vi "GetAttributeViInt32_SE_SpE_Trigger_OB.vi"(8 "error in (no error)":errorcluster {"code" format="%.0x"}, 9 "AttributeID":u32(ring)=1190055 items=["OCCUPIED_BANDWIDTH_AVERAGE_COUNT"=1190055, "OCCUPIED_BANDWIDTH_AVERAGE_MODE"=1190389, "OCCUPIED_BANDWIDTH_DETECTOR_TYPE"=1190567, "OCCUPIED_BANDWIDTH_DISPLAY_BOUNDARY_FREQUENCY_DISPLAY_TYPE"=1191461, "OCCUPIED_BANDWIDTH_DISPLAY_REF_POSITION"=1190662, "OCCUPIED_BANDWIDTH_DISPLAY_VIEW"=1191462, "OCCUPIED_BANDWIDTH_DISPLAY_VIEW_SELECTION"=1191463, "OCCUPIED_BANDWIDTH_MARKER_ACTIVE_MARKER"=1190395, "OCCUPIED_BANDWIDTH_MARKER_COUNT"=1190397, "OCCUPIED_BANDWIDTH_MARKER_DELTA_REFERENCE"=1190398, "OCCUPIED_BANDWIDTH_MARKER_TYPE"=1190568, "OCCUPIED_BANDWIDTH_POWER_REFERENCE_TYPE"=1191568, "OCCUPIED_BANDWIDTH_SWEEPCOUPLING_BANDWIDTH_SHAPE"=1190408, "OCCUPIED_BANDWIDTH_SWEEPCOUPLING_SWEEP_POINTS"=1190411, "OCCUPIED_BANDWIDTH_SWEEPCOUPLING_SWEEP_TIME_AUTO_RULES"=1190416, "OCCUPIED_BANDWIDTH_TRACE_COUNT"=1150708, "OCCUPIED_BANDWIDTH_TRACE_TYPE"=1150063, "OCCUPIED_BANDWIDTH_TRIGGER_SOURCE"=1150039, "SEMASK_AVERAGE_COUNT"=1190069, "SEMASK_DISPLAY_VIEW"=1190492, "SEMASK_DISPLAY_VIEW_SELECTION"=1150114, "SEMASK_DISPLAY_WINDOWX_REF_POSITION"=1191467, "SEMASK_DISPLAY_WINDOWY_REF_POSITION"=1190664, "SEMASK_MARKER_ACTIVE_MARKER"=1190493, "SEMASK_MARKER_COUNT"=1190495, "SEMASK_MARKER_TYPE"=1190584, "SEMASK_MEASUREMENT_TYPE"=1190475, "SEMASK_OFFSET_AVERAGE_TYPE"=1191572, "SEMASK_OFFSET_DETECTOR_TYPE"=1190508, "SEMASK_REFERENCE_CHANNEL_AVERAGE_TYPE"=1191571, "SEMASK_REFERENCE_CHANNEL_DETECTOR_TYPE"=1190485, "SEMASK_REFERENCE_CHANNEL_SWEEP_TYPE"=1191472, "SEMASK_REFERENCE_CHANNEL_SWEEP_TYPE_AUTO_RULES"=1191474, "SEMASK_SWEEPCOUPLING_BANDWIDTH_SHAPE"=1150117, "SEMASK_TRACE_COUNT"=1150710, "SEMASK_TRACE_TYPE"=1150115, "SEMASK_TRIGGER_SOURCE"=1150062, "SPECIFIC_DRIVER_CLASS_SPEC_MAJOR_VERSION"=1050515, "SPECIFIC_DRIVER_CLASS_SPEC_MINOR_VERSION"=1050516, "SPURIOUS_EMISSIONS_AVERAGE_COUNT"=1190516, "SPURIOUS_EMISSIONS_AVERAGE_MODE"=1190518, "SPURIOUS_EMISSIONS_DISPLAY_VIEW_SELECTION"=1191486, "SPURIOUS_EMISSIONS_DISPLAY_VIEW"=1190669, "SPURIOUS_EMISSIONS_MARKER_ACTIVE_MARKER"=1190523, "SPURIOUS_EMISSIONS_MARKER_COUNT"=1190525, "SPURIOUS_EMISSIONS_MARKER_DELTA_REFERENCE"=1190527, "SPURIOUS_EMISSIONS_MARKER_TYPE"=1190533, "SPURIOUS_EMISSIONS_MEASUREMENT_TYPE"=1190509, "SPURIOUS_EMISSIONS_REPORT_MODE"=1190514, "SPURIOUS_EMISSIONS_SWEEP_TIME_AUTO_RULE"=1150125, "SPURIOUS_EMISSIONS_TRIGGER_SOURCE"=1150068, "SPURIOUSEMISSIONSTRACE_COUNT"=1190614, "SWEEP_TIME_AUTO_RULES"=1191711, "SYSTEM_IO_TIMEOUT"=1191768, "TRIGGER_AIQ_MAGNITUDE_SLOPE"=1190819, "TRIGGER_EXTERNAL2_SLOPE"=1190145, "TRIGGER_EXTERNAL_SLOPE"=1190141, "TRIGGER_FRAME_SYNC_SOURCE"=1190149, "TRIGGER_FRAME_SYNCHOLDOFF_TYPE"=1150129, "TRIGGER_I_DEMODULATED_SLOPE"=1190823, "TRIGGER_INPUT_I_SLOPE"=1190827, "TRIGGER_INPUT_Q_SLOPE"=1190839, "TRIGGER_IQ_MAGNITUDE_SLOPE"=1190831, "TRIGGER_LINE_SLOPE"=1190160, "TRIGGER_Q_DEMODULATED_SLOPE"=1190835, "TRIGGER_RFBURST_LEVEL_TYPE"=1190166, "TRIGGER_RFBURST_SLOPE"=1190163, "TRIGGER_VIDEO_SLOPE"=1190170], 10 "RepCapIdentifier":string, 11 "instrument handle":refnum<k15>) -> (0 "error out":errorcluster {"code" format="%.0x"}, 2 "AttributeValue":i32, 3 "instrument handle out":refnum<k15>)   [LabVIEW 2021, in "Keysight XSAnVMA.lvlib"]
doc: "Gets Int32 Attribute from instrumrnt driver.\nThe following attributes are supported:\n\nOCCUPIED_BANDWIDTH_AVERAGE_COUNT\nOCCUPIED_BANDWIDTH_AVERAGE_MODE\nOCCUPIED_BANDWIDTH_DETECTOR_TYPE\nOCCUPIED_BANDWIDTH_DISPLAY_BOUNDARY_FREQUENCY_DISPLAY_TYPE\nOCCUPIED_BANDWIDTH_DISPLAY_REF_POSITION\nOCCUPIED_BANDWIDTH_DISPLAY_VIEW\nOCCUPIED_BANDWIDTH_DISPLAY_VIEW_SELECTION\nOCCUPIED_BANDWIDTH_MARKER_ACTIVE_MARKER\nOCCUPIED_BANDWIDTH_MARKER_COUNT\nOCCUPIED_BANDWIDTH_MARKER_DELTA_REFERENCE\nOCCUPIED_BANDWIDTH_MARKER_TYPE\nOCCUPIED_BANDWIDTH_POWER_REFERENCE_TYPE\nOCCUPIED_BANDWIDTH_SWEEPCOUPLING_BANDWIDTH_SHAPE\nOCCUPIED_BANDWIDTH_SWEEPCOUPLING_SWEEP_POINTS\nOCCUPIED_BANDWIDTH_SWEEPCOUPLING_SWEEP_TIME_AUTO_RULES\nOCCUPIED_BANDWIDTH_TRACE_COUNT\nOCCUPIED_BANDWIDTH_TRACE_TYPE\nOCCUPIED_BANDWIDTH_TRIGGER_SOURCE\nSEMASK_AVERAGE_COUNT\nSEMASK_DISPLAY_VIEW\nSEMASK_DISPLAY_VIEW_SELECTION\nSEMASK_DISPLAY_WINDOWX_REF_POSITION\nSEMASK_DISPLAY_WINDOWY_REF_POSITION\nSEMASK_MARKER_ACTIVE_MARKER\nSEMASK_MARKER_COUNT\nSEMASK_MARKER_TYPE\nSEMASK_MEASUREMENT_TYPE\nSEMASK_OFFSET_AVERAGE_TYPE\nSEMASK_OFFSET_DETECTOR_TYPE\nSEMASK_REFERENCE_CHANNEL_AVERAGE_TYPE\nSEMASK_REFERENCE_CHANNEL_DETECTOR_TYPE\nSEMASK_REFERENCE_CHANNEL_SWEEP_TYPE\nSEMASK_REFERENCE_CHANNEL_SWEEP_TYPE_AUTO_RULES\nSEMASK_SWEEPCOUPLING_BANDWIDTH_SHAPE\nSEMASK_TRACE_COUNT\nSEMASK_TRACE_TYPE\nSEMASK_TRIGGER_SOURCE\nSPECIFIC_DRIVER_CLASS_SPEC_MAJOR_VERSION\nSPECIFIC_DRIVER_CLASS_SPEC_MINOR_VERSION\nSPURIOUS_EMISSIONS_AVERAGE_COUNT\nSPURIOUS_EMISSIONS_AVERAGE_MODE\nSPURIOUS_EMISSIONS_DISPLAY_VIEW_SELECTION\nSPURIOUS_EMISSIONS_DISPLAY_VIEW\nSPURIOUS_EMISSIONS_MARKER_ACTIVE_MARKER\nSPURIOUS_EMISSIONS_MARKER_COUNT\nSPURIOUS_EMISSIONS_MARKER_DELTA_REFERENCE\nSPURIOUS_EMISSIONS_MARKER_TYPE\nSPURIOUS_EMISSIONS_MEASUREMENT_TYPE\nSPURIOUS_EMISSIONS_REPORT_MODE\nSPURIOUS_EMISSIONS_SWEEP_TIME_AUTO_RULE\nSPURIOUS_EMISSIONS_TRIGGER_SOURCE\nSPURIOUSEMISSIONSTRACE_COUNT\nSWEEP_TIME_AUTO_RULES\nSYSTEM_IO_TIMEOUT\nTRIGGER_AIQ_MAGNITUDE_SLOPE\nTRIGGER_EXTERNAL2_SLOPE\nTRIGGER_EXTERNAL_SLOPE\nTRIGGER_FRAME_SYNC_SOURCE\nTRIGGER_FRAME_SYNCHOLDOFF_TYPE\nTRIGGER_FRAME_RFBURST_SLOPE\nTRIGGER_I_DEMODULATED_SLOPE\nTRIGGER_INPUT_I_SLOPE\nTRIGGER_INPUT_Q_SLOPE\nTRIGGER_IQ_MAGNITUDE_SLOPE\nTRIGGER_LINE_SLOPE\nTRIGGER_Q_DEMODULATED_SLOPE\nTRIGGER_RFBURST_LEVEL_TYPE\nTRIGGER_RFBURST_SLOPE\nTRIGGER_VIDEO_SLOPE"
uses:
  <instrlib>/Keysight XSAnVMA/Keysight XSAnVMA.lvlib
  KtXSAnVMA_64.dll
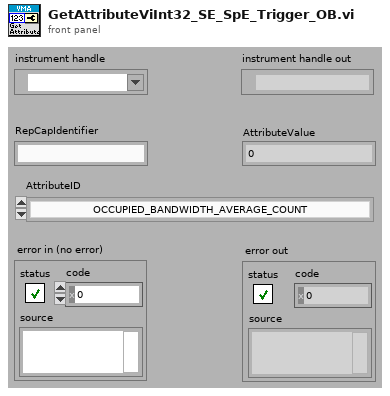
[diagram p1: front panel]
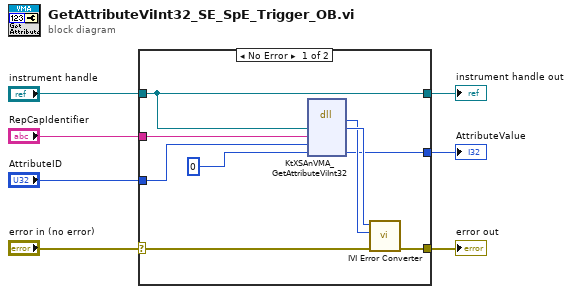
[diagram p0: block diagram]
diagram:
  n1 = case shown="No Error" "error in (no error)" {
    selector: "error in (no error)" -> [w14 w18]
    tunnel: [w13 w18] -> w7
    tunnel: "instrument handle" -> [w8 w17]
    tunnel: "RepCapIdentifier" -> [w12 _]
    tunnel: "AttributeID" -> [w11 _]
    tunnel: [w9 _] -> w3
    tunnel: [w8 w17] -> w2
    frame No Error {
      n2 = dll-call lib="KtXSAnVMA**.dll" fn="KtXSAnVMA_GetAttributeViInt32"("Vi"=w8, "RepCapIdentifier"=w12, "AttributeID"=w11, "AttributeValue"=0) -> ("return type"=w15:i32, "Vi"=w16:u32, "AttributeValue"=w9:i32)  [unwired: 5 in, 2 out]
      n3 = call <instrlib>:"IVI Error Converter.vi"("error in (no error)"=w14, "IVI error code (0)"=w15, "instrument handle"=w16) -> ("error out"=w13:errorcluster)  [unwired: 7 in, 1 out]
    }
    frame Error {
    }
  }
  "error out" <- w7
  "instrument handle out" <- w2
  "AttributeValue" <- w3
